vi "Run Bfr Rx - CachedSize - Copy Cache.vi"(7 "External Buffer":u64 format="%016x", 8 "error in (no error)":errorcluster, 11 "Cached Buffer in":T1 {"Cache Buffer" format="%016x"}) -> (0 "error out":errorcluster, 3 "Cached Buffer out":T1 {"Cache Buffer" format="%016x"})   [LabVIEW 2021, in "UDP-Custom-Device Engine.lvlib"]
uses:
  UDP-Custom-Device Engine.lvlib
  Types/Engine - Buffered Rx Cached Buffer.ctl
  <vilib>/NI VeriStand/VeriStand Data/Pointer Operations/Pointer.In-Place Read (1D U8).vi
  <vilib>/NI VeriStand/VeriStand Data/Pointer Operations/Pointer.Write (1D U8).vi
  <vilib>/NI VeriStand/VeriStand Data/VeriStand Data.lvlib
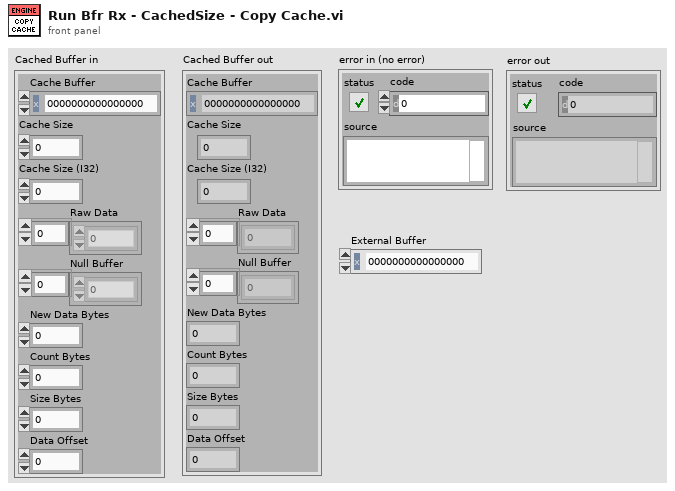
[diagram p1: front panel]
types:
  T1 = typedef "UDP-Custom-Device Engine.lvlib/Engine - Buffered Rx Cached Buffer.ctl" = cluster{"Cache Buffer":u64, "Cache Size":u64, "Cache Size (I32)":i32, "Raw Data":u8[], "Null Buffer":u8[], "New Data Bytes":u64, "Count Bytes":u64, "Size Bytes":u64, "Data Offset":u64}
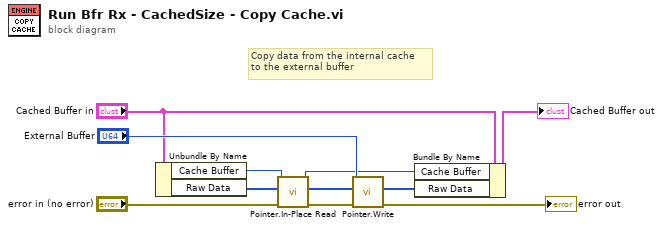
[diagram p0: block diagram]
diagram:
  # "Copy data from the internal cache\nto the external buffer"
  n1 = Unbundle By Name("Cached Buffer in") -> ("Cache Buffer"=w6:u64, "Raw Data"=w7:u8[])
  n2 = call-poly <vilib>:"Pointer.In-Place Read.vi"("error in (no error)"="error in (no error)", "allocated array in"=w7, "pointer in"=w6) -> ("error out"=w11:errorcluster, "array out"=w10:u8[], "pointer out"=w4:u64)  [unwired: 6 in]
  n3 = call-poly <vilib>:"Pointer.Write.vi"("error in (no error)"=w11, "values"=w10, "pointer in"="External Buffer") -> ("error out"=→"error out":errorcluster, "values out"=w3:u8[])  [unwired: 6 in, 1 out]
  n4 = Bundle By Name(cluster="Cached Buffer in", "Cache Buffer"=w4, "Raw Data"=w3) -> (→"Cached Buffer out":T1)
